vi "Init PLC Settings.vi"(8 "error in":errorcluster, 11 "queue in":refnum<queue>) -> (0 "error out":errorcluster, 3 "queue out":refnum<queue>)   [LabVIEW 2018]
uses:
  Ctls/QueueData.ctl
  Ctls/State.ctl
  Ctls/CmdData.ctl
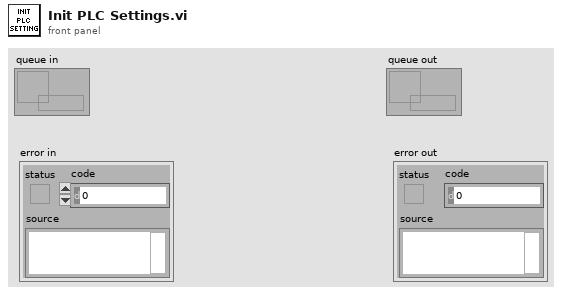
[diagram p1: front panel]
types:
  T1 = typedef "CmdData.ctl" = cluster{"Address Areas":u8, "Data Block #":u16, "Start Address (bytes)":u32, "Write Data Float":sgl, "Bit #":u16, "Write Data Boolean":bool}
  T2 = typedef "State.ctl" = enum16{"poll data command", "display update", "init", "send bool command", "send float command", "datalog", "error", "fix rating rpm 1", "fix rating rpm 2", "fix both rating rpm", "fix rating rpm all", "terminate", "log Motor Speed Setting"}
  T3 = typedef "QueueData.ctl" = cluster{"State":T2, "Command Data":T1}
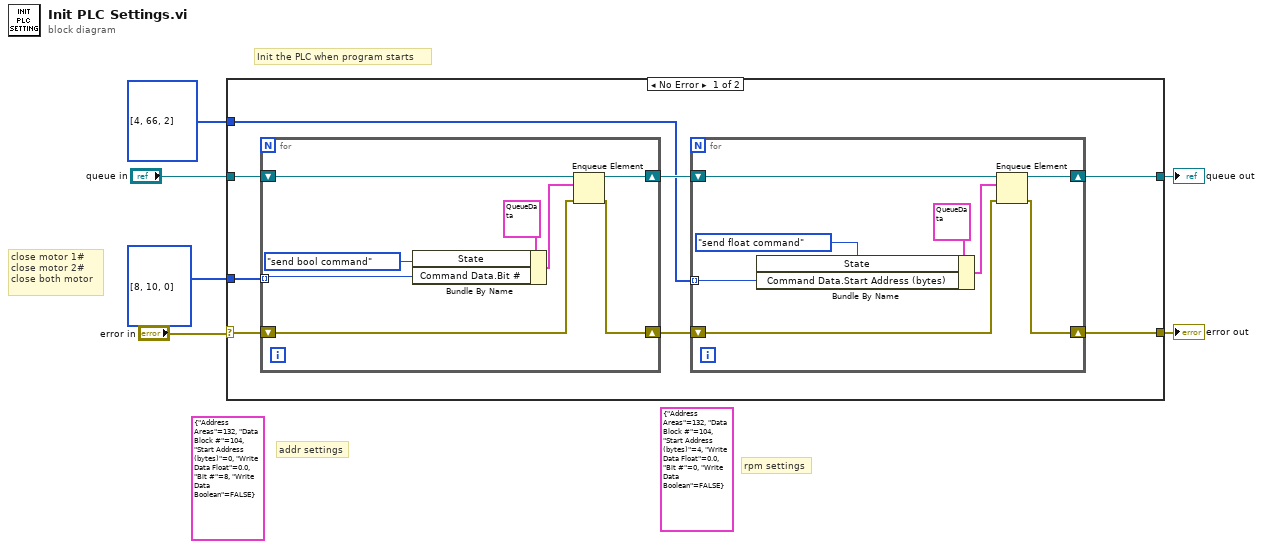
[diagram p0: block diagram]
diagram:
  (unwired) T1 {"Address Areas"=132, "Data Block #"=104, "Start Address (bytes)"=4, "Write Data Float"=0.0, "Bit #"=0, "Write Data Boolean"=FALSE} ("Command Data")
  (unwired) T1 {"Address Areas"=132, "Data Block #"=104, "Start Address (bytes)"=0, "Write Data Float"=0.0, "Bit #"=8, "Write Data Boolean"=FALSE} ("Command Data")
  # "rpm settings"
  # "Init the PLC when program starts"
  # "addr settings"
  # "close motor 1# \nclose motor 2#\nclose both motor"
  n1 = case shown="No Error" "error in" {
    selector: "error in" -> [w12 w31]
    tunnel: "queue in" -> [w13 w32]
    tunnel: u16[] [8, 10, 0] -> [w14 _]
    tunnel: [w9 w32] -> w3
    tunnel: [w8 w31] -> w2
    tunnel: u32[] [4, 66, 2] -> [w7 _]
    frame No Error {
      n2 = for {
        tunnel: w14 -> [w23] mode=indexing
        shift-right: [w27] -> w11
        shift-left: w13 -> [w28]
        shift-right: [w24] -> w10
        shift-left: w12 -> [w25]
        n3 = Bundle By Name(cluster=T3 {"State"=enum."init", "Command Data"={"Address Areas"=132, "Data Block #"=104, "Start Address (bytes)"=0, "Write Data Float"=0.0, "Bit #"=0, "Write Data Boolean"=FALSE}} ("QData"), "State"=State."send bool command", "Command Data.Bit #"=w23) -> (w26:T3)
        n4 = Enqueue Element(queue=w28, element=w26, error in (no error)=w25) -> (queue out=w27:refnum<queue>, error out=w24:errorcluster)  [unwired: 1 in, 1 out]
      }
      n5 = for {
        shift-right: [w19] -> w9
        shift-left: w11 -> [w20]
        shift-right: [w16] -> w8
        shift-left: w10 -> [w17]
        tunnel: w7 -> [w15] mode=indexing
        n6 = Bundle By Name(cluster=T3 {"State"=enum."init", "Command Data"={"Address Areas"=132, "Data Block #"=104, "Start Address (bytes)"=4, "Write Data Float"=0.0, "Bit #"=0, "Write Data Boolean"=FALSE}} ("QData"), "State"=State."send float command", "Command Data.Start Address (bytes)"=w15) -> (w18:T3)
        n7 = Enqueue Element(queue=w20, element=w18, error in (no error)=w17) -> (queue out=w19:refnum<queue>, error out=w16:errorcluster)  [unwired: 1 in, 1 out]
      }
    }
    frame Error {
    }
  }
  "queue out" <- w3
  "error out" <- w2
